vi "Size.vi"(8 "error in (no error)":errorcluster, 11 "Generic Array Data in":refnum<class "Generic Array Data.lvclass">) -> (0 "error out":errorcluster, 2 "Size":i32, 3 "Generic Array Data out":refnum<class "Generic Array Data.lvclass">)   [LabVIEW 2020, in "Data.lvlib" / "Generic Array Data.lvclass"]
doc: "Return the size of the generic data element."
uses:
  Generic Array Data.lvclass
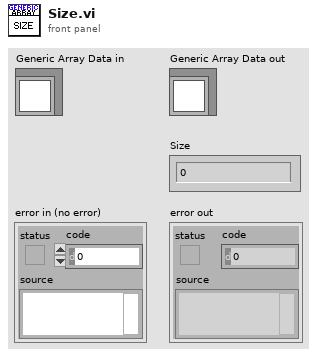
[diagram p1: front panel]
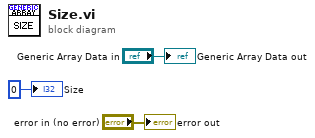
[diagram p0: block diagram]
diagram:
  "error out" <- "error in (no error)"
  "Generic Array Data out" <- "Generic Array Data in"
  "Size" <- 0 ("Size")
